vi "Principal Component Analysis.vi"() -> ()   [LabVIEW 2023]
doc: "This example shows how to perform principal components analysis on a multivariate time series with the TSA Principal Component Analysis VI.\n\n<b>Instructions:</b>\n1) Run this VI.\n2) Compare the variance of each channel before and after PCA."
uses:
  <vilib>/addons/Time Series Analysis/Utilities.llb/TSA Data.ctl
  <vilib>/addons/Time Series Analysis/Statistical Analysis.llb/TSA Principal Component Analysis (Waveform).vi
  <vilib>/addons/_Advanced Signal Processing/NI_AdvSigProcTSA.lvlib
panel:
  in  "stop":bool
  out "Correlation Plot 2":cluster{"Y":dbl[], "Y":dbl[]}(graph)
  out "Correlation Plot 1":cluster{"Y":dbl[], "Y":dbl[]}(graph)
  out "Two Channel Vibration Data":waveform(dbl)[](graph)
  out "Principal Components Scores":waveform(dbl)[](graph)
  # "Overview: Shows how to perform principal components analysis on a multivariate time series with the TSA Principal Component Analysis VI.\nRequirements: LabVIEW Full Development System, Advanced Signal Processing Toolkit\nInstructions: \n1. Run this VI.\n2. Compare the variance of each channel before and after PCA.\n3.  Click Stop to stop the VI."
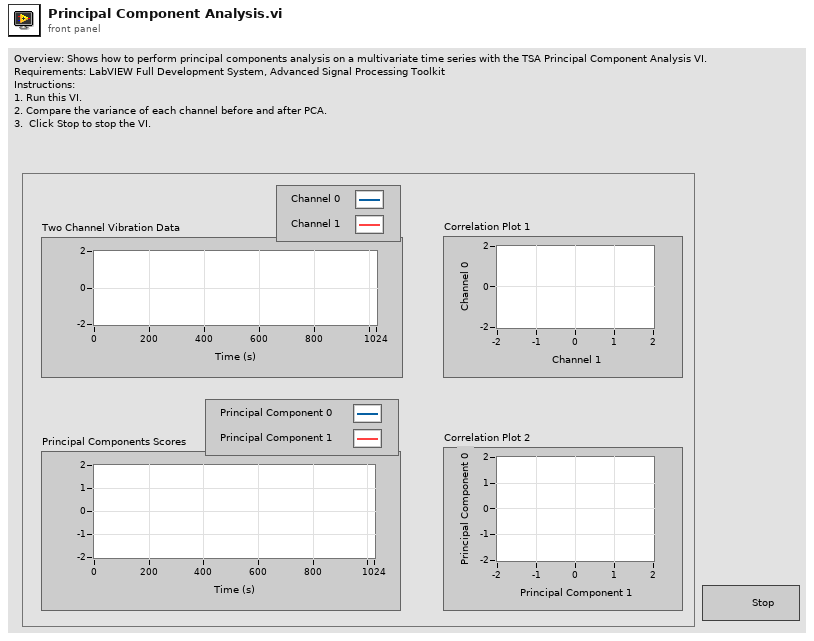
[diagram p1: front panel]
types:
  T1 = typedef "NI_AdvSigProcTSA.lvlib/TSA Data.ctl" = u16
  T2 = cluster{"Signal out":waveform(dbl), "Signal out":waveform(dbl)}
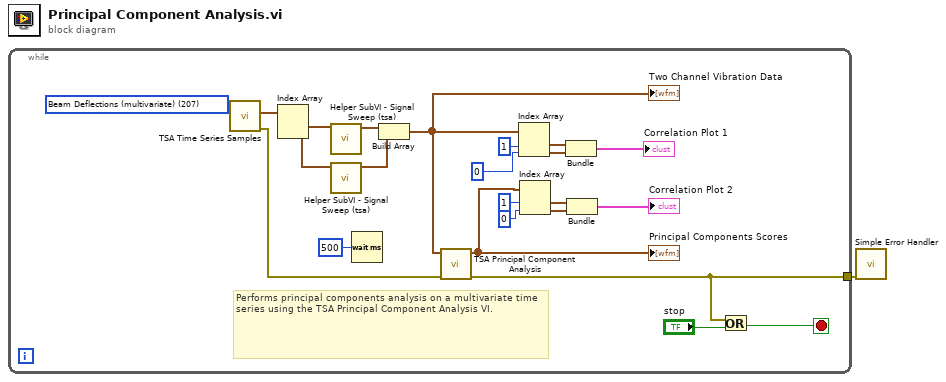
[diagram p0: block diagram]
diagram:
  n1 = while {
    tunnel: [w2] -> w1
    stop <- w18 stop-if-true
    w10 = T1 207 items=["Kobe Earthquake"=201, "EEG"=210, "Bearing Vibration (simulated)"=211, "Period Product Sales"=214, "Beam Vibration (nonlinear)"=217, "Beam Vibration (linear)"=218, "Signal With Echo"=219, "Engine Knocking"=220, "Power Line"=221, "-"=200, "Beam Deflections (multivariate)"=207, "Structure Vibration (multivariate)"=208, "Human MEG (multivariate)"=222] ("data")
    # "Performs principal components analysis on a multivariate time series using the TSA Principal Component Analysis VI."
    n2 = call <vilib>:"TSA Time Series Samples.vi"("data"=w10) -> ("error out"=w3:errorcluster, "multivariate time series"=w16:waveform(dbl)[])  [unwired: 1 in, 8 out]
    n3 = Index Array(array=w16) -> (element #1=w15:waveform(dbl), element #2=w14:waveform(dbl))  [unwired: 2 in]
    n4 = call "Helper SubVI - Signal Sweep (tsa).vi"("Signal in"=w15) -> ("Signal out"=w13:waveform(dbl))  [unwired: 10 in]
    n5 = call "Helper SubVI - Signal Sweep (tsa).vi"("Signal in"=w14) -> ("Signal out"=w11:waveform(dbl))  [unwired: 10 in]
    n6 = Wait (ms)(milliseconds to wait=u32 500 ("millisecond multiple")) -> ()  [unwired: 1 out]
    n7 = Build Array(w13, w11) -> (w12:waveform(dbl)[])
    "Two Channel Vibration Data" <- w12
    n8 = call-poly <vilib>:"TSA Principal Component Analysis.vi"("error in (no error)"=w3, "Xt"=w12) -> ("error out"=w2:errorcluster, "Xt out"=w24:waveform(dbl)[])  [unwired: 1 in, 7 out]
    "Principal Components Scores" <- w24
    n9 = Index Array(array=w12, index #1=1 ("index (row)"), index #2=0 ("index (row)")) -> (element #1=w5:waveform(dbl), element #2=w4:waveform(dbl))
    n10 = Index Array(array=w24, index #1=1 ("index (row)"), index #2=0 ("index (row)")) -> (element #1=w7:waveform(dbl), element #2=w6:waveform(dbl))
    n11 = Bundle("Signal out"=w5, "Signal out"=w4) -> (→"Correlation Plot 1":T2)  [unwired: 1 out]
    n12 = Bundle("Xt"=w7, "Xt"=w6) -> (→"Correlation Plot 2":cluster{"Xt":waveform(dbl), "Xt":waveform(dbl)})  [unwired: 1 out]
    n13 = Or(x=w2, y="stop") -> (x .or. y?=w18:bool)
  }
  n14 = call <vilib>:"Simple Error Handler.vi"("error in (no error)"=w1) -> ()  [unwired: 1 in, 8 out]
